vi "specu1a 1.0.0 Open Target Device.vi"(3 "error in":errorcluster, 5 "Unit ID":string) -> (0 "error out":errorcluster, 1 "Unit ID copy":string, 2 "Device Handle":i32)   [LabVIEW 2019]
uses:
  specu1a.dll
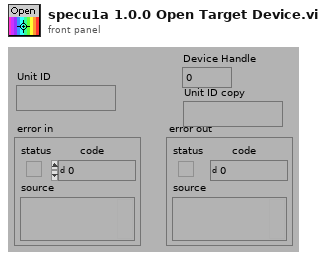
[diagram p1: front panel]
types:
  T1 = typedef "specu1a 1.0.0 Error codes.ctl" = enum16{"INVALID_HANDLE_VALUE", "USBDEV_SUCCESS", "USBDEV_INVALID_HANDLE", "USBDEV_UNSUCCESS", "USBDEV_INVALID_VALUE", "USBDEV_CHECK_NORMAL", "USBDEV_CHECK_INVALID", "USBDEV_CHECK_REMOVE", "USBDEV_CHECK_OTHER", "USBDEV_RESET_ERROR", "USBDEV_BULKSIZE_ERROR", "USBDEV_BULK_READ_ERROR", "USBDEV_BULK_NOT_UPDATED", "USBDEV_TIME_OVER_ERROR", "USBDEV_TIME_UNDER_ERROR", "USBDEV_TIME_SET_ERROR", "USBDEV_SET_GAIN_ERROR", "USBDEV_GET_TEMP_ERROR", "USBDEV_SET_TRIGGER_ERROR", "USBDEV_RW_EEP_ADDR_ERROR", "USBDEV_RW_EEP_SIZE_ERROR", "USBDEV_RW_EEP_OVER_ERROR", "USBDEV_RW_EEP_ERROR", "UNITID_PRODUCTID_CONFLICT", "UNKNOWN_ERROR"}
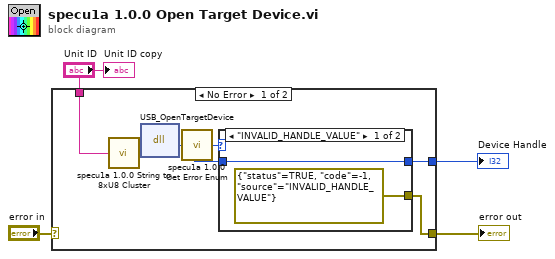
[diagram p0: block diagram]
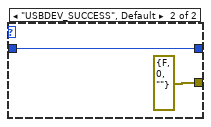
[diagram p2: hidden frame]
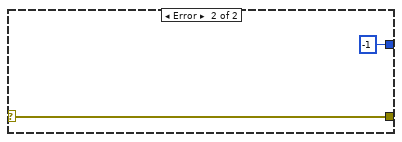
[diagram p3: hidden frame]
diagram:
  n1 = case shown="No Error" "error in" {
    selector: "error in" -> [_ w16]
    tunnel: [w10 w16] -> w4
    tunnel: [w9 -1 ("Device Handle")] -> w3
    tunnel: "Unit ID" -> [w5 _]
    frame No Error {
      n2 = call "specu1a 1.0.0 String to 8xU8 Cluster.vi"("String in"=w5) -> ("8xU8 Cluster"=w7:cluster{u8, u8, u8, u8, u8, u8, u8, u8})  [unwired: 14 in]
      n3 = dll-call lib="C:/Users/martzlab/Desktop/SIO 179/Nitrate/64/EvaluationSoftware/minispec labview/Hamamatsu Spectrometer Dll/specu1a.dll" fn="USB_OpenTargetDevice" label="1.0.0 Open Target Device"("8xU8 Cluster"=w7) -> ("Device Handle"=w6:i32)  [unwired: 4 in, 2 out]
      n4 = call "specu1a 1.0.0 Get Error Enum.vi"("Error Code in"=w6) -> ("Specu1a 1.0.0 Error code out"=w8:T1)  [unwired: 4 in]
      n5 = case shown="\"INVALID_HANDLE_VALUE\"" w8 {
        tunnel: [w11 w13] -> w9
        tunnel: [errorcluster {"status"=TRUE, "code"=-1, "source"="INVALID_HANDLE_VALUE"} ("error out") errorcluster {"status"=FALSE, "code"=0, "source"=""} ("error out")] -> w10
        tunnel: w6 -> [w11 w13]
        frame "INVALID_HANDLE_VALUE" {
        }
        frame "USBDEV_SUCCESS", Default {
        }
      }
    }
    frame Error {
    }
  }
  "error out" <- w4
  "Device Handle" <- w3
  "Unit ID copy" <- "Unit ID"
